vi "MathScript.vi"(11 "x":dbl[](array[numeric])=[1.0, 2.0, 3.0]) -> (1 "y(1) in MathScript Node":dbl, 2 "y(1) in LabVIEW":dbl, 3 "y":dbl[](array[numeric]))   [LabVIEW 2019]
doc: "Demonstrates some fundamental concepts associated with the MathScript Node."
uses:
  <vilib>/imath/engines/lvmath/Plug In/_Char/NIMS_CH_character datatype.ctl
  <vilib>/imath/engines/lvmath2/RunTimeEngine/IndexRead/NIMS V(S).vi
  <instcachedir>/0/NIMS V(S)_0488751826AF41519A22953C041130DC.lvgen/NIMS V(S)_0488751826AF41519A22953C041130DC_000.vi
  <vilib>/imathl/engines/lvmath/Functions/Error Handling/Create Error.vi
  <vilib>/imath/engines/lvmath2/RunTimeEngine/BuiltInFunctions/dot/NIMS_dot(GV,GV).vi
  <instcachedir>/0/NIMS_dot(GV,GV)_B9FAA411F4494E9B94D442721014A3FA.lvgen/NIMS_dot(GV,GV)_B9FAA411F4494E9B94D442721014A3FA_000.vi
  <vilib>/imath/engines/lvmath2/RunTimeEngine/ErrorHandling/NIMS_Error From Error Code.vi
  <vilib>/imath/engines/lvmath2/RunTimeEngine/NodeEndStatement/NIMS_NodeEndStatement_Output.vi
  <instcachedir>/0/NIMS_NodeEndStatement_Output_53EC0D466D134D7ABD903AC30B43404B.lvgen/NIMS_NodeEndStatement_Output_53EC0D466D134D7ABD903AC30B43404B_001.vi
  <instcachedir>/0/NIMS_NodeEndStatement_Output_53EC0D466D134D7ABD903AC30B43404B.lvgen/NIMS_NodeEndStatement_Output_53EC0D466D134D7ABD903AC30B43404B_005.vi
  <vilib>/imath/engines/lvmath2/RunTimeEngine/ErrorHandling/NIMS_Finalize Error.vi
  <vilib>/imath/engines/lvmath2/RunTimeEngine/BuiltInFunctions/rand/NIMS_rand(1,I32).vi
  <vilib>/imath/engines/lvmath2/RunTimeEngine/BuiltInFunctions/rand/NIMS_rand(I32,I32).vi
  <vilib>/imath/engines/lvmath2/RunTimeEngine/RowToken/NIMS_RowToken_M_M.vi
  <instcachedir>/0/NIMS_RowToken_M_M_5745C4A5DE4D41039F822F7C59AEBB94.lvgen/NIMS_RowToken_M_M_5745C4A5DE4D41039F822F7C59AEBB94_004.vi
  <vilib>/imath/engines/lvmath/Functions/Error Handling/MergeErrorsWrapper.vi
  <vilib>/imath/engines/lvmath2/RunTimeEngine/BuiltInFunctions/ones/NIMS_V=ones(I32,I32).vi
  <vilib>/imath/engines/lvmath2/RunTimeEngine/ArithmeticOperatorToken/NIMS_ArithmeticOperator_times.vi
  <instcachedir>/0/NIMS_ArithmeticOperator_times_BC2A7BF92F8245379E8C6B3F6BDCD4B7.lvgen/NIMS_ArithmeticOperator_times_BC2A7BF92F8245379E8C6B3F6BDCD4B7_008.vi
  <vilib>/imath/engines/lvmath2/RunTimeEngine/RangeToken/NIMS_Range_R2 - Integer.vi
  <instcachedir>/0/NIMS_Range_R2 - Integer_5118B3908D7D4A9BA0DEB8EE73549D2D.lvgen/NIMS_Range_R2 - Integer_5118B3908D7D4A9BA0DEB8EE73549D2D_000.vi
  <vilib>/imath/engines/lvmath2/RunTimeEngine/CommandStatement/MC_CommandStatement_break.vi
  <vilib>/imath/engines/lvmath2/RunTimeEngine/BuiltInFunctions/randnormal/NIMS_randnormal(1,I32).vi
  <vilib>/imath/engines/lvmath2/RunTimeEngine/BuiltInFunctions/findnz/NIMS_[1o]_findnz(GColV).vi
  <instcachedir>/0/NIMS_[1o]_findnz(GColV)_FDE4D4C48C0F4A35B030964F2F22918F.lvgen/NIMS_[1o]_findnz(GColV)_FDE4D4C48C0F4A35B030964F2F22918F_000.vi
  <vilib>/imath/engines/lvmath2/RunTimeEngine/RowToken/NIMS_RowToken_CV_CV.vi
  <instcachedir>/0/NIMS_RowToken_CV_CV_3D6C8EEAD808447A8CA3C46EB7EFCD94.lvgen/NIMS_RowToken_CV_CV_3D6C8EEAD808447A8CA3C46EB7EFCD94_002.vi
  <vilib>/imath/engines/lvmath2/RunTimeEngine/MatrixToken/NIMS_MatrixToken_M_M.vi
  <instcachedir>/0/NIMS_MatrixToken_M_M_E7822903E2DE4826A718AD6172B79999.lvgen/NIMS_MatrixToken_M_M_E7822903E2DE4826A718AD6172B79999_005.vi
  <vilib>/imath/engines/lvmath2/RunTimeEngine/ErrorHandling/NIMS_Create Error From Enums.vi
  <vilib>/imath/engines/lvmath2/RunTimeEngine/IndexRead/NIMS V(V).vi
  <instcachedir>/0/NIMS V(V)_298D9CB7BFEB42B8BC8D9C3C28AE8C70.lvgen/NIMS V(V)_298D9CB7BFEB42B8BC8D9C3C28AE8C70_000.vi
  <vilib>/imath/engines/lvmath2/RunTimeEngine/IndexReplace/NIMS V(V)=V.vi
  <instcachedir>/0/NIMS V(V)=V_03D9C6F13D634C4EA430E227ADCC6F66.lvgen/NIMS V(V)=V_03D9C6F13D634C4EA430E227ADCC6F66_000.vi
  <vilib>/imath/engines/lvmath2/RunTimeEngine/ArithmeticOperatorToken/NIMS_ArithmeticOperator_plus.vi
  <instcachedir>/0/NIMS_ArithmeticOperator_plus_A857F7369B7D4E138264023AAAB8243E.lvgen/NIMS_ArithmeticOperator_plus_A857F7369B7D4E138264023AAAB8243E_004.vi
  <vilib>/imath/engines/lvmath2/RunTimeEngine/IndexRead/NIMS M($,V).vi
  <instcachedir>/0/NIMS M($,V)_706F2CE2C8E141269FD4C8A402E169C5.lvgen/NIMS M($,V)_706F2CE2C8E141269FD4C8A402E169C5_004.vi
  <vilib>/imath/engines/lvmath2/RunTimeEngine/BuiltInFunctions/sum/NIMS_sum(GM,Sca).vi
  <instcachedir>/0/NIMS_sum(GM,Sca)_C7E3CBE1717D47E9BA3F6C65B3FF862B.lvgen/NIMS_sum(GM,Sca)_C7E3CBE1717D47E9BA3F6C65B3FF862B_001.vi
  <vilib>/imath/engines/lvmath2/RunTimeEngine/ArithmeticOperatorToken/NIMS_ArithmeticOperator_minus.vi
  <instcachedir>/0/NIMS_ArithmeticOperator_minus_A2D45F688BFF4915B286240799BA2370.lvgen/NIMS_ArithmeticOperator_minus_A2D45F688BFF4915B286240799BA2370_003.vi
  <instcachedir>/0/NIMS_ArithmeticOperator_times_BC2A7BF92F8245379E8C6B3F6BDCD4B7.lvgen/NIMS_ArithmeticOperator_times_BC2A7BF92F8245379E8C6B3F6BDCD4B7_000.vi
  <vilib>/imath/engines/lvmath/Plug In/_Char/NIMS_CH_Character RV to String.vi
  <vilib>/imath/engines/lvmath2/RunTimeEngine/IndexRead/NIMS M($,S).vi
  <instcachedir>/0/NIMS M($,S)_3E5749BBB62E49528D4765A77F1F6D98.lvgen/NIMS M($,S)_3E5749BBB62E49528D4765A77F1F6D98_002.vi
  <vilib>/imath/engines/lvmath2/RunTimeEngine/BuiltInFunctions/plot/NIMS_plot(RM, RM, Str).vi
panel:
  out "Dot Product":dbl
  # "x^2"
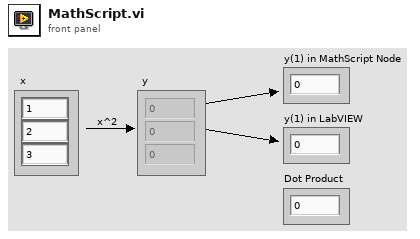
[diagram p1: front panel]
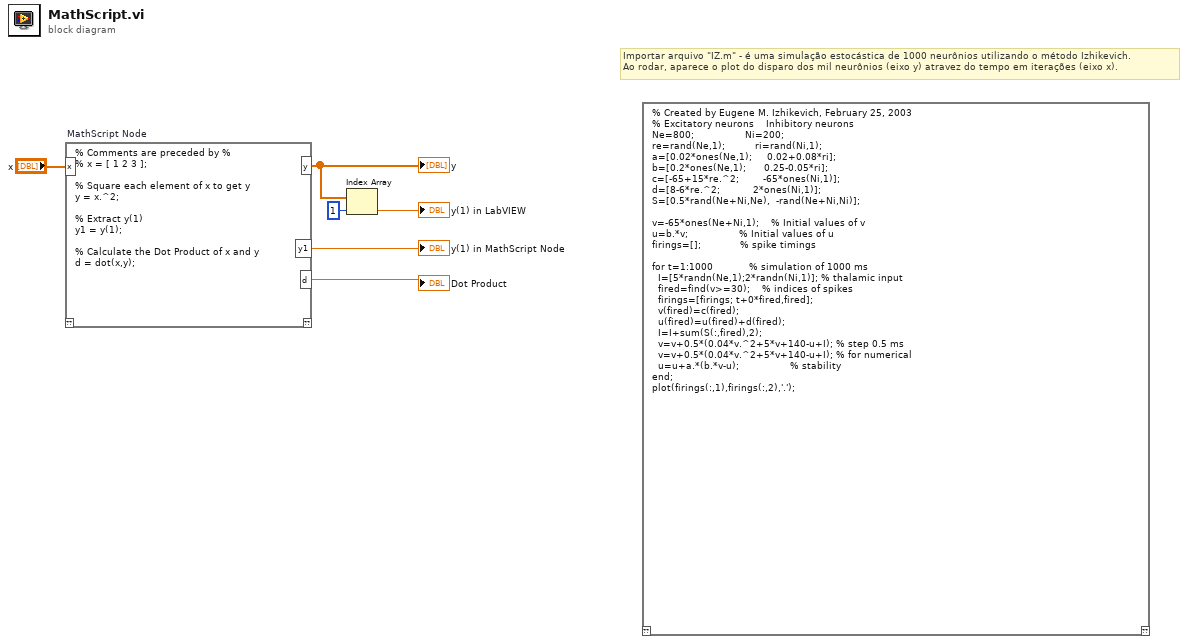
[diagram p0: block diagram]
diagram:
  # "Importar arquivo \"IZ.m\" - é uma simulação estocástica de 1000 neurônios utilizando o método Izhikevich.\nAo rodar, aparece o plot do disparo dos mil neurônios (eixo y) atravez do tempo em iterações (eixo x)."
  n1 = mathscript code="% Comments are preceded by %\n% x = [ 1 2 3 ];\n\n% Square each element of x to get y\ny = x.^2;\n\n% Extract y(1)\ny1 = y(1);\n\n% Calculate the Dot Product of x and y\nd = dot(x,y);"("x"="x") -> ("y"=w4:dbl[], "y1"=→"y(1) in MathScript Node":dbl, "d"=→"Dot Product":dbl)  [unwired: 1 in, 1 out]
  "y" <- w4
  n2 = Index Array "Index Array"(array=w4, index=1) -> (element=→"y(1) in LabVIEW":dbl)
  n3 = mathscript code="% Created by Eugene M. Izhikevich, February 25, 2003\n% Excitatory neurons    Inhibitory neurons\nNe=800;                 Ni=200;\nre=rand(Ne,1);          ri=rand(Ni,1);\na=[0.02*ones(Ne,1);     0.02+0.08*ri];\nb=[0.2*ones(Ne,1);      0.25-0.05*ri];\nc=[-65+15*re.^2;        -65*ones(Ni,1)];\nd=[8-6*re.^2;           2*ones(Ni,1)];\nS=[0.5*rand(Ne+Ni,Ne),  -rand(Ne+Ni,Ni)];\n\nv=-65*ones(Ne+Ni,1);    % Initial values of v\nu=b.*v;                 % Initial values of u\nfirings=[];             % spike timings\n\nfor t=1:1000            % simulation of 1000 ms\n  I=[5*randn(Ne,1);2*randn(Ni,1)]; % thalamic input\n  fired=find(v>=30);    % indices of spikes\n  firings=[firings; t+0*fired,fired];\n  v(fired)=c(fired);\n  u(fired)=u(fired)+d(fired);\n  I=I+sum(S(:,fired),2);\n  v=v+0.5*(0.04*v.^2+5*v+140-u+I); % step 0.5 ms\n  v=v+0.5*(0.04*v.^2+5*v+140-u+I); % for numerical\n  u=u+a.*(b.*v-u);                 % stability\nend;\nplot(firings(:,1),firings(:,2),'.');"() -> ()  [unwired: 1 in, 1 out]
